vi "matlab code example.vi"() -> ()   [LabVIEW 2010]
panel:
  in  "exit":bool
  out "Notes 2":string="Update MyCsvFileName.csv with your file name.\n\nThe data will be stored on the variable matrix.data.\n\nTo check the number of lines of the matrix, use:\n   length(matrix.data)"
  in  "Copy 2":bool
  in  "Matlab code to import the CSV file created 2":string="matrix = importdata('MyCsvFileName.csv');"
  out "Notes":string="Update MyCsvFileName.csv with your file name.\n\nThe data will be stored on the variable matrix.\n\nTo check the number of lines of the matrix, use:\n   length(matrix)"
  in  "Copy":bool
  in  "Matlab code to import the CSV file created":string="matrix = csvread('MyCsvFileName.csv',1,0);"
  # "Matlab code to import the CSV file created -- Option 1\n(Slower)"
  # "Matlab code to import the CSV file created -- Option 2\n(Faster but only works when all the lines of the CSV file are using the same number of columns)"
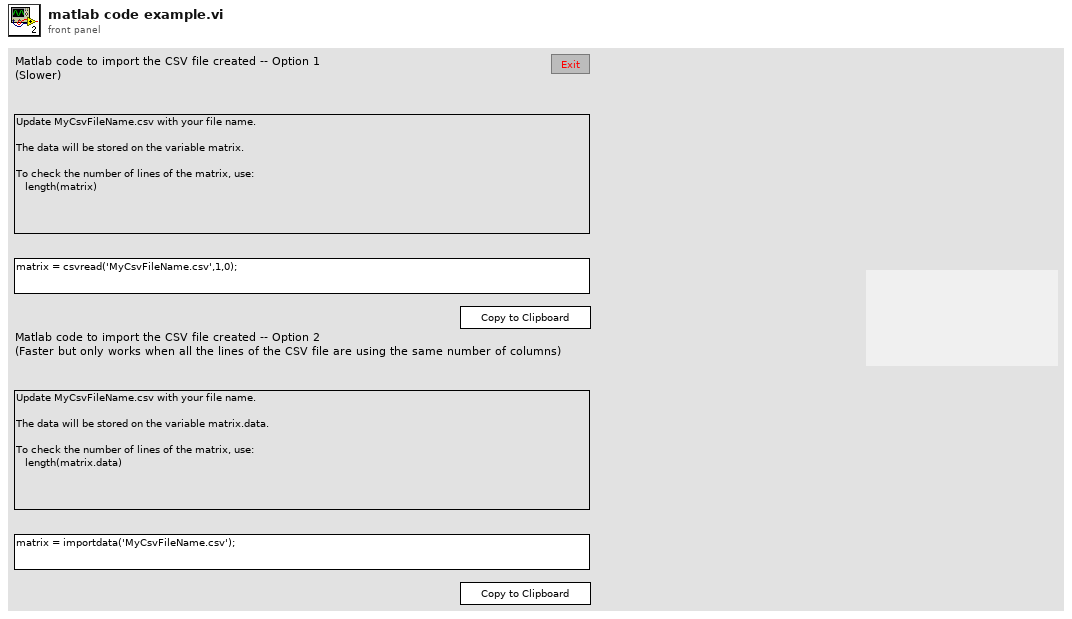
[diagram p1: front panel]
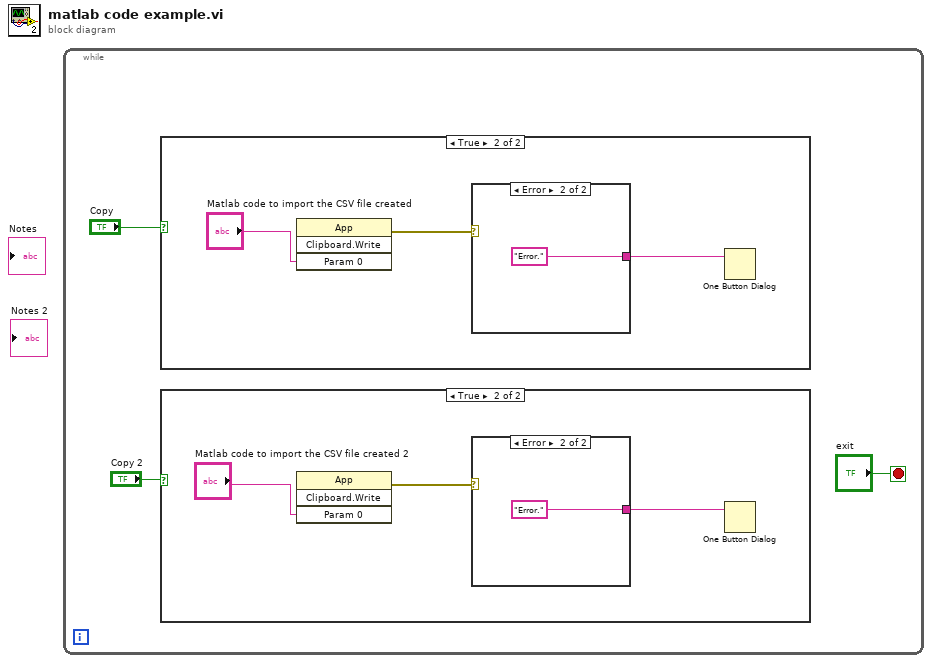
[diagram p0: block diagram]
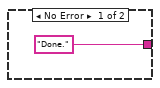
[diagram p3: hidden frame]
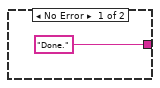
[diagram p5: hidden frame]
diagram:
  n1 = while {
    stop <- "exit" stop-if-true
    n2 = case shown="True" "Copy" {
      frame False {
      }
      frame True {
        n3 = invoke class="App" method="Clipboard.Write"("Param 0"="Matlab code to import the CSV file created") -> (error out=w10:errorcluster)  [unwired: 3 in, 3 out]
        n4 = case shown="Error" w10 {
          tunnel: ["Done." ("message") "Error." ("message")] -> w9
          frame No Error {
          }
          frame Error {
          }
        }
        n5 = One Button Dialog(message=w9) -> ()  [unwired: 1 in, 1 out]
      }
    }
    n6 = case shown="True" "Copy 2" {
      frame False {
      }
      frame True {
        n7 = invoke class="App" method="Clipboard.Write"("Param 0"="Matlab code to import the CSV file created 2") -> (error out=w6:errorcluster)  [unwired: 3 in, 3 out]
        n8 = case shown="Error" w6 {
          tunnel: ["Done." ("message") "Error." ("message")] -> w5
          frame No Error {
          }
          frame Error {
          }
        }
        n9 = One Button Dialog(message=w5) -> ()  [unwired: 1 in, 1 out]
      }
    }
  }
